vi "Autonomous Independent.vi"() -> ()   [LabVIEW 2015]
doc: "This VI is called when autonomous begins, and will automatically be terminated when autonomous ends. You can carry out timed or sensor driven robot movement independently without needing to return to the caller."
uses:
  <vilib>/Rock Robotics/WPI/Utilities/WPI_GetSetVariantRefNum.vi
  <vilib>/Rock Robotics/Network Tables/NT Read String.vi
  <vilib>/Rock Robotics/Network Tables/NT Write Numeric Array.vi
  <vilib>/Rock Robotics/Network Tables/NT Write Number.vi
  <vilib>/addons/control/pid/pid.llb/PID (DBL).vi
  Robot Global Data.vi
  <vilib>/Rock Robotics/Network Tables/NT Read Number.vi
  <vilib>/addons/control/pid/NI_PID_pid.lvlib
  navX Library v2/navX Library v2.lvlib
panel:
  in  "Roll":dbl
  in  "Angle":dbl
  in  "Distance":dbl=120.0
  in  "Task":u16(ring) items=["Forward", "Backward", "Turn", "Shoot", "Turn Angle", "Roll G", "Roll L"]
  in  "Aiming Gains":T1={"proportional gain (Kc)"=1.0, "integral time (Ti, min)"=0.01, "derivative time (Td, min)"=0.0} {"derivative time (Td, min)" format="%.3f"; "integral time (Ti, min)" format="%.3f"; "proportional gain (Kc)" format="%.3f"}
  out "Yaw":dbl(graph)
  in  "Target Angle":dbl=30.0
  out "E1 Rate":dbl
  out "E2 Rate":dbl
  out "Yaw Display":dbl
  in  "Single Turn Gains":T1={"proportional gain (Kc)"=0.12, "integral time (Ti, min)"=0.0, "derivative time (Td, min)"=0.0} {"derivative time (Td, min)" format="%.3f"; "integral time (Ti, min)" format="%.3f"; "proportional gain (Kc)" format="%.3f"}
  in  "Yaw":T1={"proportional gain (Kc)"=0.2, "integral time (Ti, min)"=0.0, "derivative time (Td, min)"=0.0} {"derivative time (Td, min)" format="%.3f"; "integral time (Ti, min)" format="%.3f"; "proportional gain (Kc)" format="%.3f"}
  out "Right Motor Speed":dbl(graph)
  out "Left Motor Speed":dbl(graph)
  out "Right Motor":dbl(graph)
  out "Left Motor":dbl(graph)
  in  "Distance":dbl=120.0
  in  "Speed Gains":T1={"proportional gain (Kc)"=0.65, "integral time (Ti, min)"=0.001, "derivative time (Td, min)"=0.001} {"derivative time (Td, min)" format="%.3f"; "integral time (Ti, min)" format="%.3f"; "proportional gain (Kc)" format="%.3f"}
  out "E2 Dist":dbl
  out "E1 Dist":dbl
  # "Be sure to right-click and choose Data Operations>>Make Current Value default if you want to save the array values with the VI"
  # "Encoder Distance Traveled"
  # "Speed we are assigning the motors and Encoder Rate"
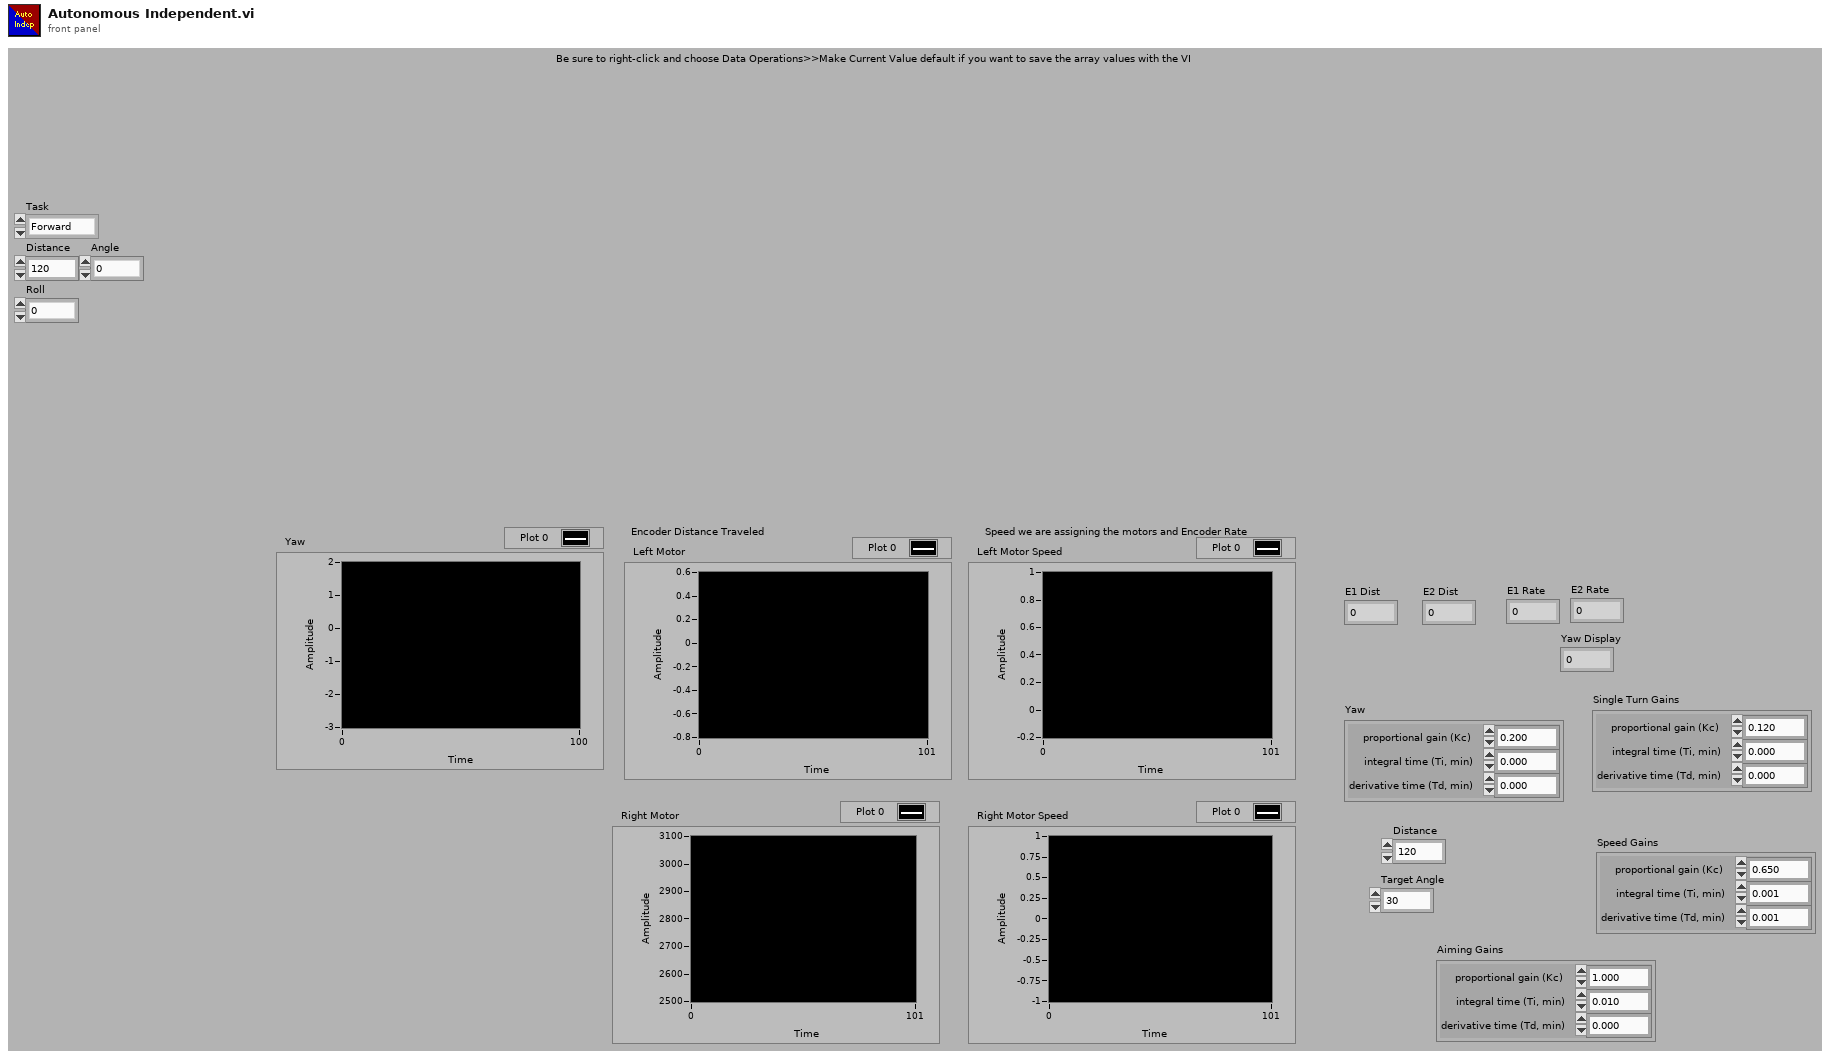
[diagram p1: front panel]
types:
  T1 = cluster{"proportional gain (Kc)":dbl, "integral time (Ti, min)":dbl, "derivative time (Td, min)":dbl}
  T2 = typedef "WPI_JoystickDevRef.ctl" = cluster{"Device":T3}
  T3 = typedef "WPI_JoystickDeviceEnum.ctl" = enum16{"USB 0", "USB 1", "USB 2", "USB 3", "USB 4", "USB 5"}
  T4 = typedef "navX Library v2.lvlib/Z900_navX_DeviceTypeDef.ctl" = cluster{"Interface":cluster{"Protocol":T5, "Update Rate (4Hz-60Hz)":u8, "navX Open TypeDef":variant}, "Notify Packet":refnum<notifier>, "Loop VI Refnum":refnum<vi>, "Ready to Close Occurrence Refnum":refnum<k4>}
  T5 = typedef "navX Library v2.lvlib/Z900_navX_ProtocolTypeDef.ctl" = enum16{"SERIAL", "I2C", "SPI"}
  T6 = typedef "WPI_EncoderDevRef.ctl" = cluster{"DevStatus":errorcluster, "EncoderIndex":T7, "CounterIndex":T8, "DistancePerCount":dbl, "Decoding Type":T9}
  T7 = typedef "FPGA_EncoderIdx.ctl" = enum8{"Enc 0", "Enc 1", "Enc 2", "Enc 3", "Enc 4", "Enc 5", "Enc 6", "Enc 7", "Invalid"}
  T8 = typedef "FPGA_CounterCtrSystemIndex.ctl" = enum8{"Ctr 0", "Ctr 1", "Ctr 2", "Ctr 3", "Ctr 4", "Ctr 5", "Ctr 6", "Ctr 7", "Invalid"}
  T9 = typedef "WPI_EncoderType.ctl" = enum16{"1x", "2x", "4x"}
  T10 = cluster{"Yaw":dbl, "Roll":dbl, "Pitch":dbl, "Heading":dbl, "Fused Heading":dbl}
  T11 = typedef "WPI_RobotDriveDevRef.ctl" = cluster{"DevStatus":errorcluster, "Motors[]":T12[], "Square Inputs":bool, "Max Output":dbl}
  T12 = typedef "WPI_MotorControlDeviceRef.ctl" = cluster{"DeviceStatus":errorcluster, "Type":T13, "PWM":cluster{"PWM Channel":T14, "DeadBand":T15}, "CAN":cluster{"Device Number":u8, "Control Mode":T16, "Semaphore":T17, "Max Vout":dbl, "TalonSRX Control Mode":T18}, "Invert":bool}
  T13 = typedef "WPI_MotorControlType.ctl" = enum16{"PWM", "CAN", "CANTalonSRX"}
  T14 = typedef "FPGA_DIOPWMChannel.ctl" = enum8{"PWM 0", "PWM 1", "PWM 2", "PWM 3", "PWM 4", "PWM 5", "PWM 6", "PWM 7", "PWM 8", "PWM 9", "PWM MXP 0", "PWM MXP 1", "PWM MXP 2", "PWM MXP 3", "PWM MXP 4", "PWM MXP 5", "PWM MXP 6", "PWM MXP 7", "PWM MXP 8", "PWM MXP 9", "Invalid"}
  T15 = typedef "WPI_PWMDeadband.ctl" = cluster{"Name":string, "maxPositivePwm":i32, "minPositivePwm":i32, "centerPwm":i32, "maxNegativePwm":i32, "minNegativePwm":i32, "angularRange":u16}
  T16 = typedef "WPI_CANJaguar_ControlMode.ctl" = enum8{"Percent VBus", "Current", "Speed", "Position", "Voltage"}
  T17 = typedef "Semaphore RefNum" = refnum<k1>
  T18 = typedef "WPI_CANTalonSRX_APIControlMode.ctl" = enum8{"Percent VBus", "Speed", "Position", "Slave", "Unchanged / Invalid", "Voltage Compensation", "Current", "Motion Profile"}
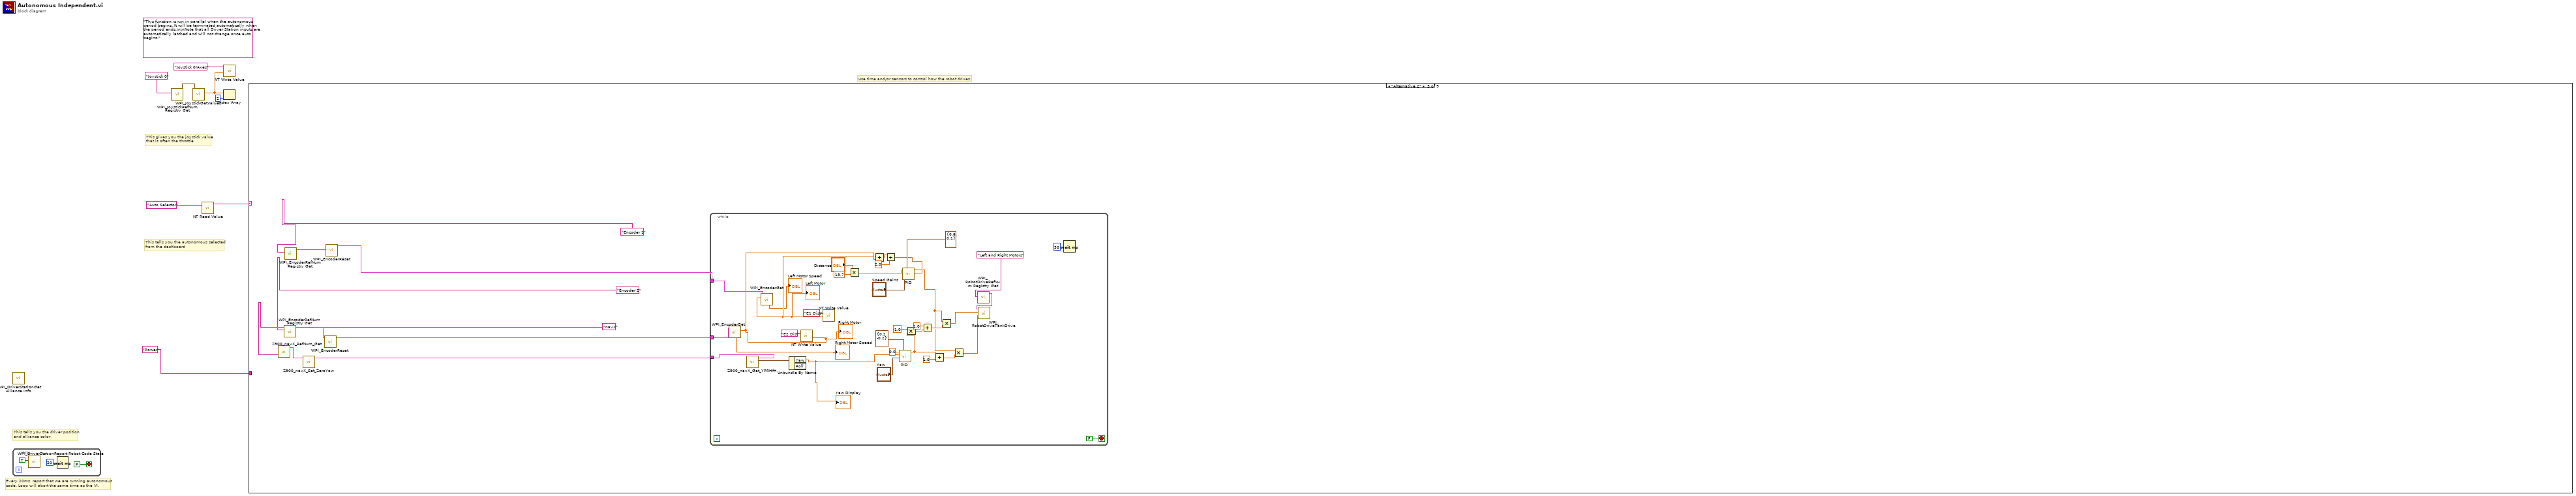
[diagram p0: block diagram]
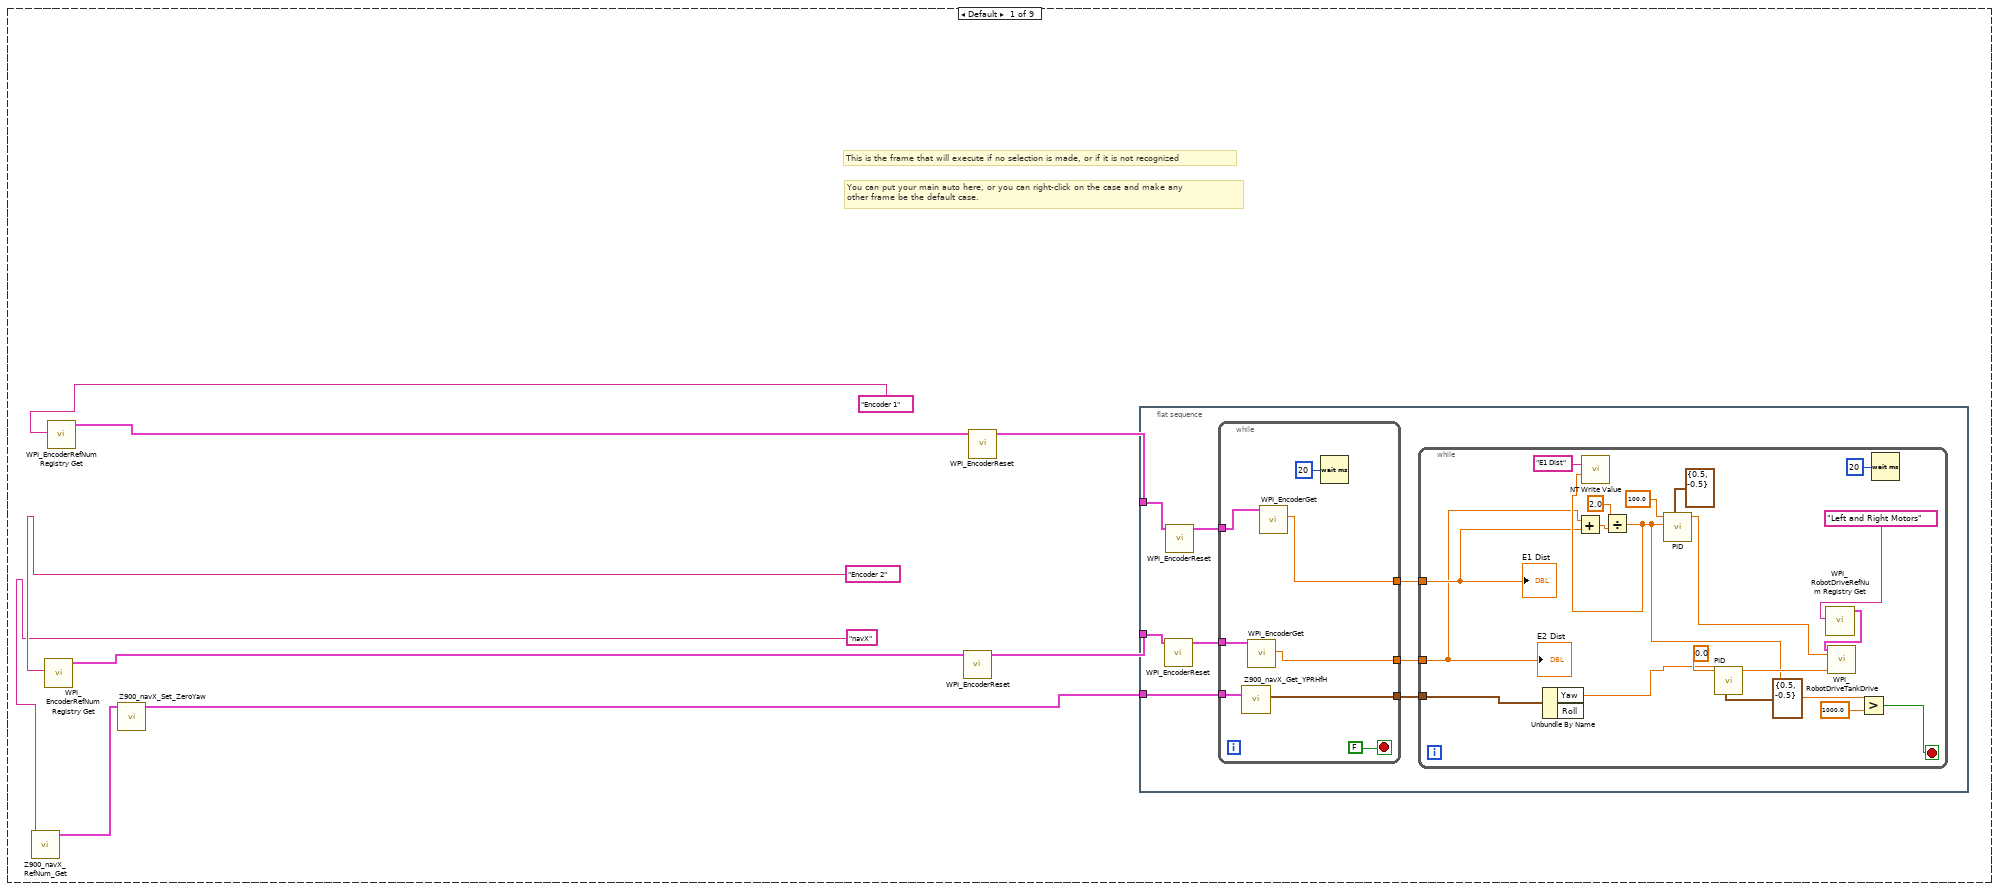
[diagram p2: hidden frame]
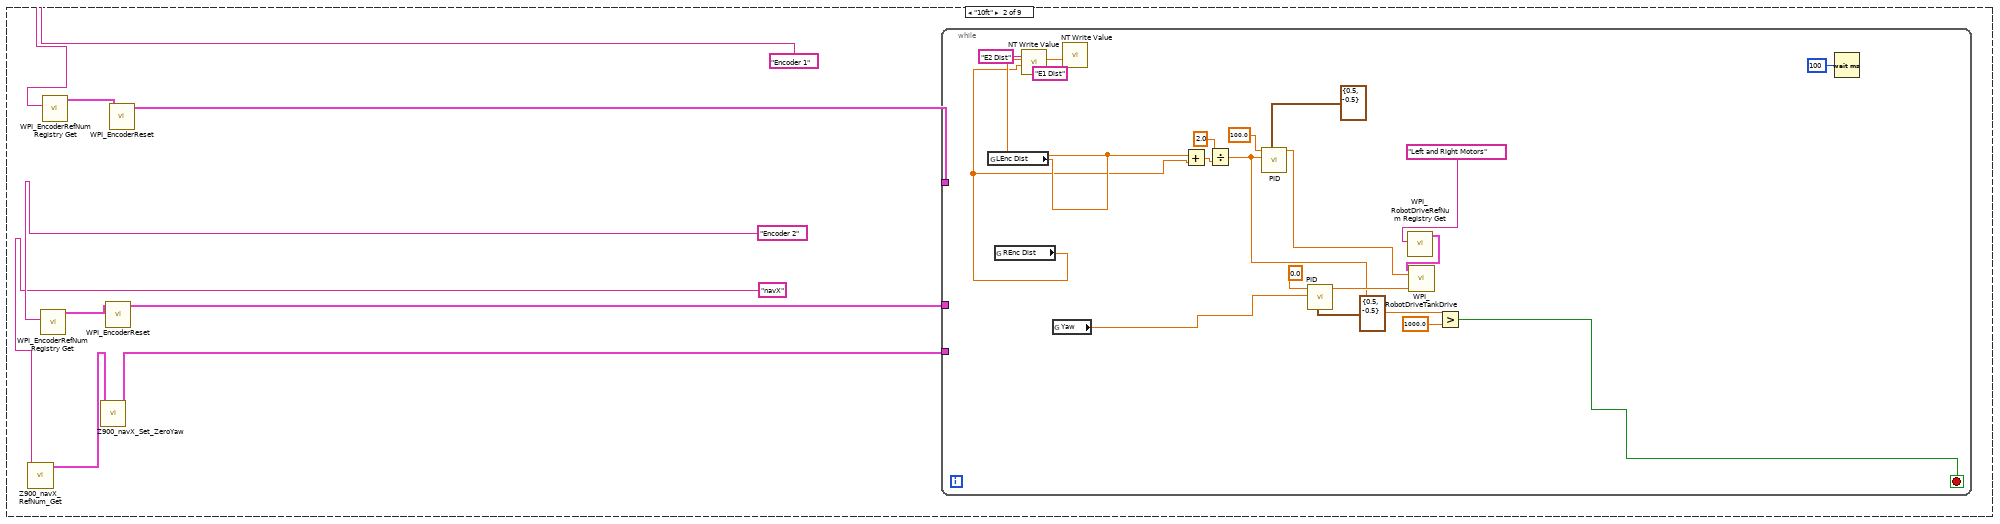
[diagram p3: hidden frame]
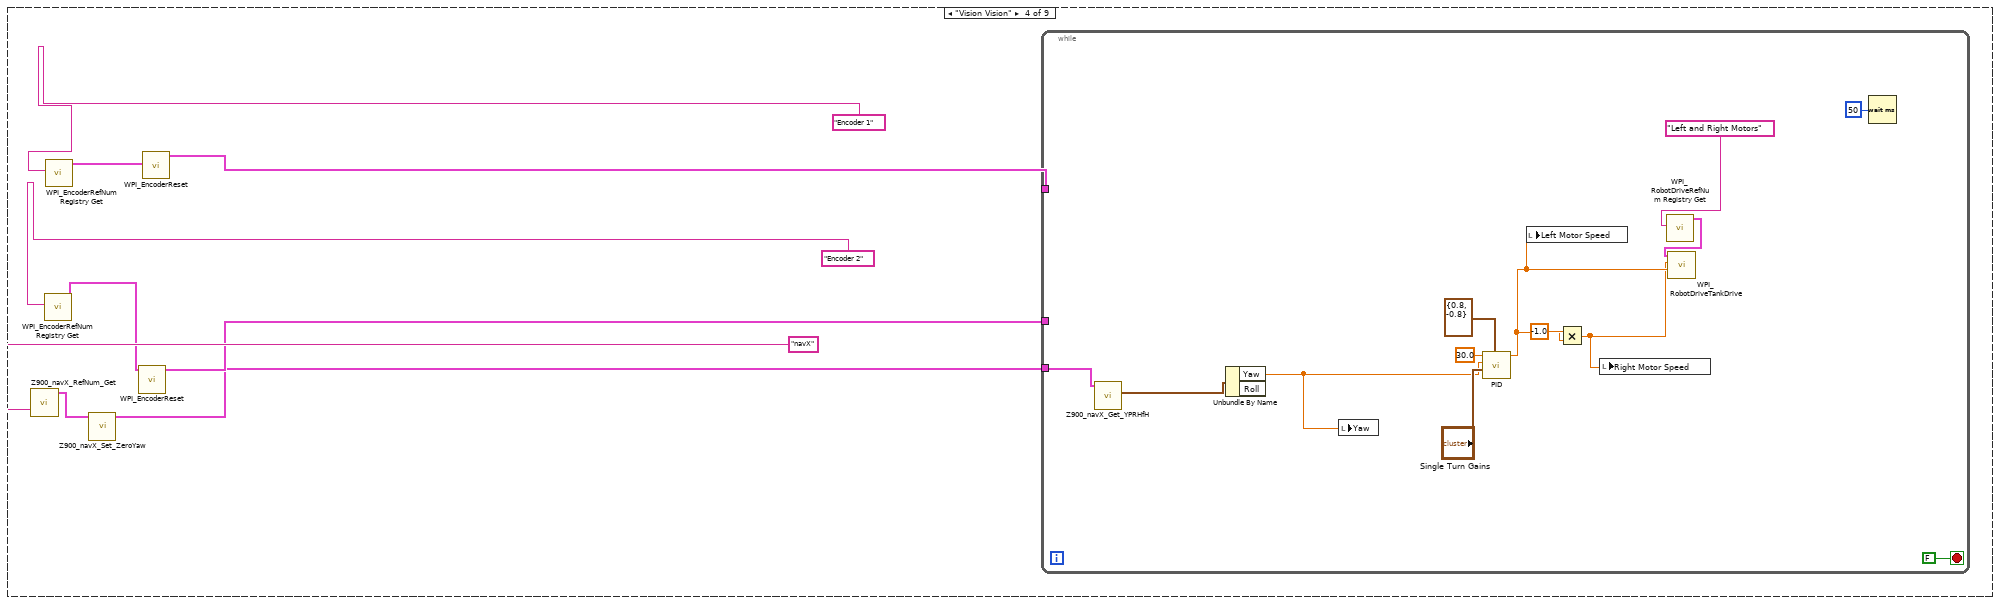
[diagram p4: hidden frame]
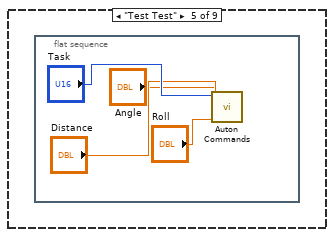
[diagram p5: hidden frame]
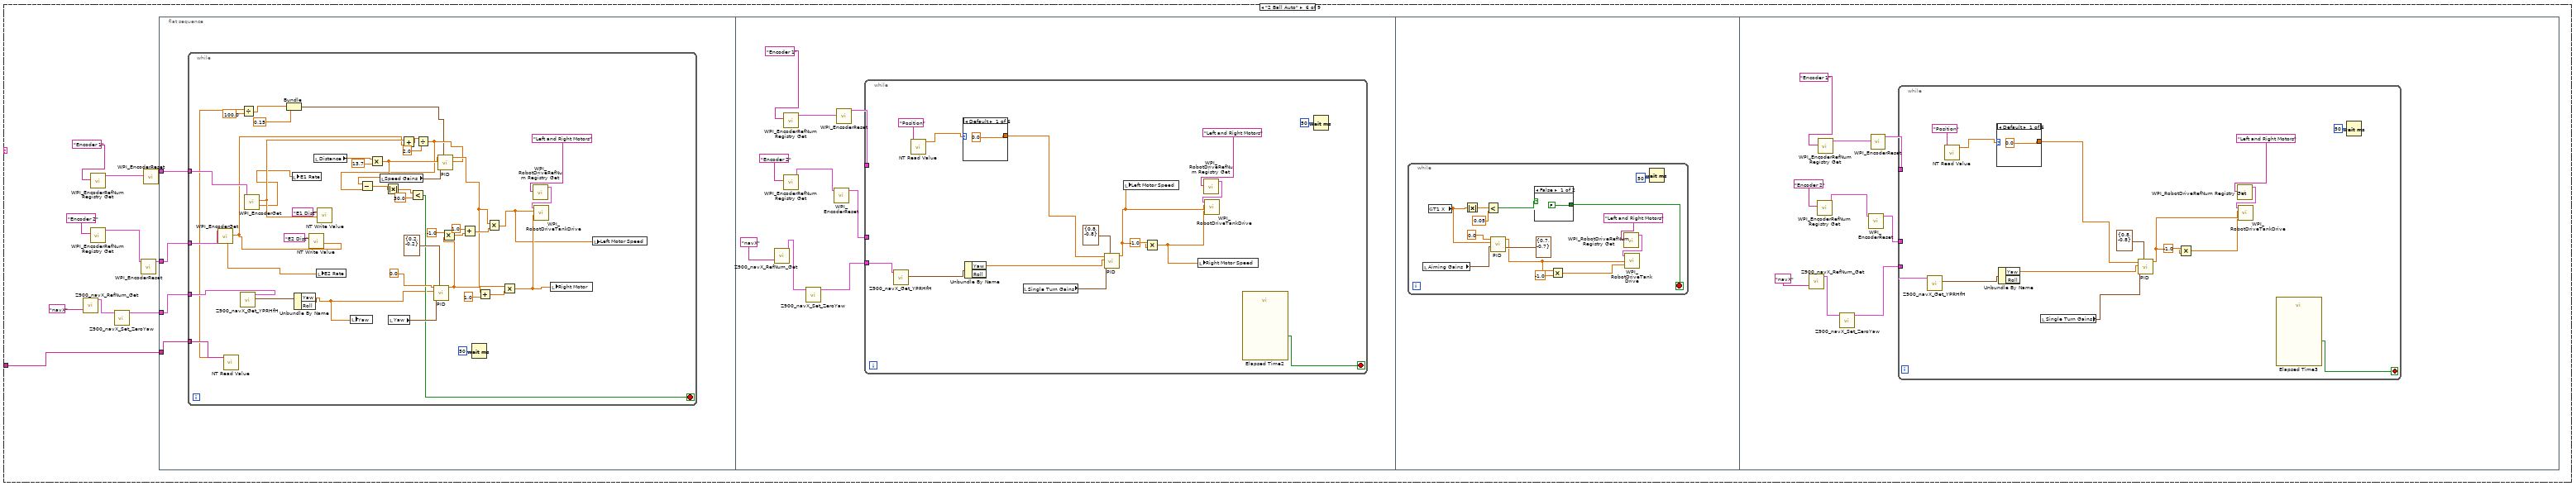
[diagram p6: hidden frame]
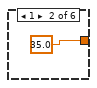
[diagram p7: hidden frame]
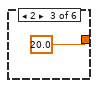
[diagram p8: hidden frame]
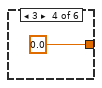
[diagram p9: hidden frame]
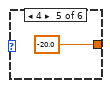
[diagram p10: hidden frame]
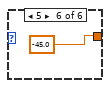
[diagram p11: hidden frame]
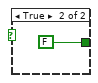
[diagram p12: hidden frame]
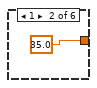
[diagram p13: hidden frame]
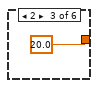
[diagram p14: hidden frame]
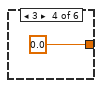
[diagram p15: hidden frame]
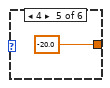
[diagram p16: hidden frame]
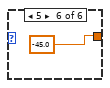
[diagram p17: hidden frame]
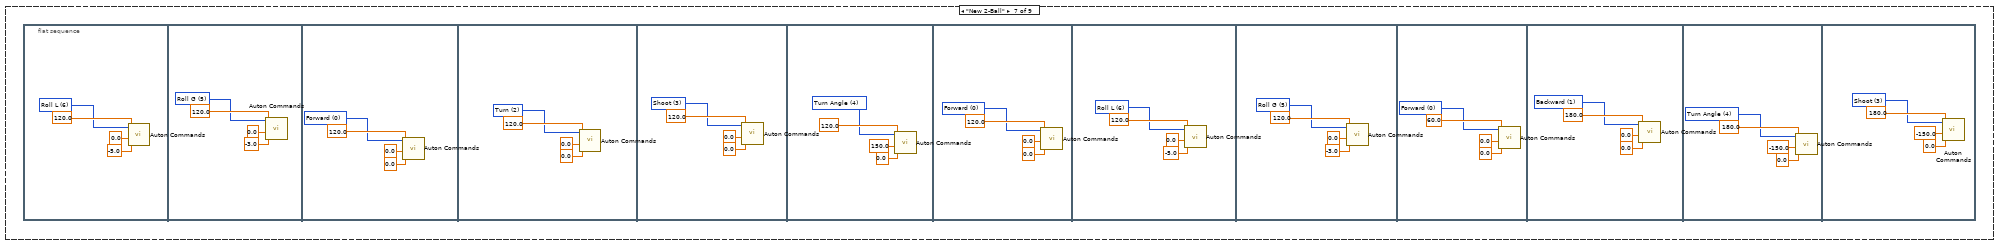
[diagram p18: hidden frame]
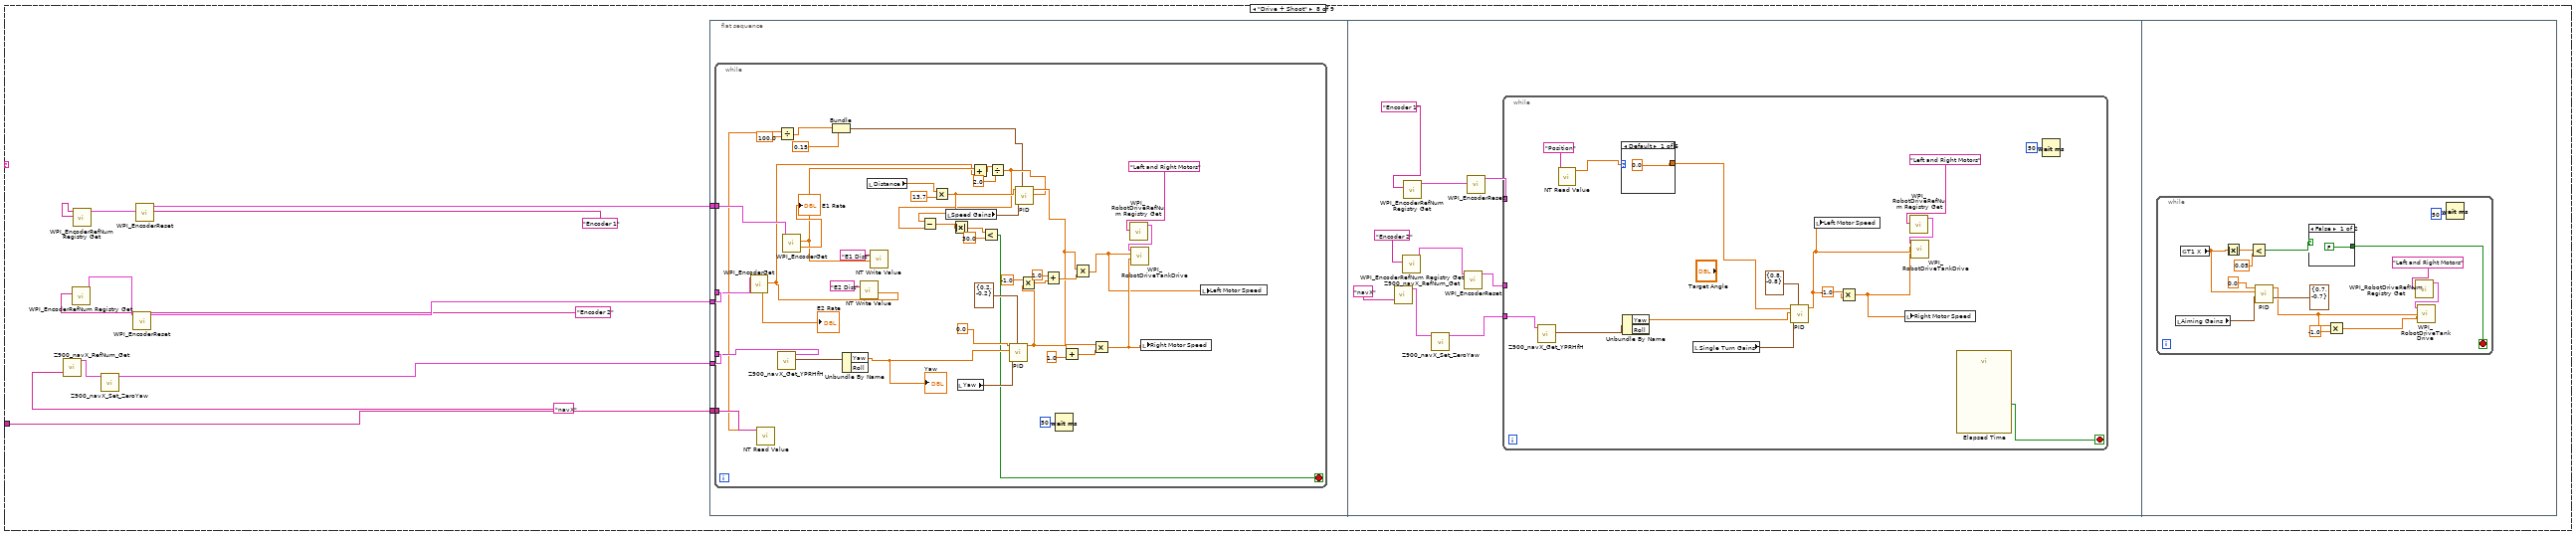
[diagram p19: hidden frame]
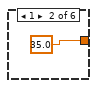
[diagram p20: hidden frame]
diagram:
  (unwired) "This function is run in parallel when the autonomous period begins. It will be terminated automatically when the period ends.\n\nNote that all Driver Station inputs are automatically latched and will not change once auto begins."
  # "This tells you the autonomous selected\nfrom the dashboard"
  # "Every 20ms, report that we are running autonomous\ncode. Loop will abort the same time as the VI."
  # "This gives you the joystick value\nthat is often the throttle"
  # "Use time and/or sensors to control how the robot drives."
  # "This tells you the driver position\nand alliance color"
  n1 = while {
    stop <- FALSE stop-if-true
    n2 = call <vilib>:"WPI_DriverStationReport Robot Code State.vi"("Autonomous"=TRUE) -> ()  [unwired: 10 in, 1 out]
    n3 = Wait (ms)(milliseconds to wait=u32 20) -> ()  [unwired: 1 out]
  }
  n4 = call <vilib>:"WPI_DriverStationGet Alliance Info.vi"() -> ()  [unwired: 12 out]
  n5 = call <vilib>:"WPI_JoystickRefNum Registry Get.vi"("refnum name"="Joystick 0") -> ("JoystickDevRef"=w7:T2)  [unwired: 1 in, 9 out]
  n6 = call <vilib>:"WPI_JoystickGetValues.vi"("JoystickDevRef"=w7) -> ("Axes"=w3:dbl[])  [unwired: 6 in, 4 out]
  n7 = call-poly <vilib>:"NT Read Value.vi"("Name"="Auto Selector") -> ("String"=w4:string)  [unwired: 9 in, 1 out]
  n8 = call-poly <vilib>:"NT Write Value.vi"("Numeric Array"=w3, "Name"="Joystick 0/Axes") -> ()  [unwired: 9 in, 1 out]
  n9 = Index Array(array=w3, index=2) -> ()  [unwired: 1 out]
  n10 = case shown="\"Alternative 2\"" w4 {
    tunnel: "Power" ("Name") -> [_ _ _ _ _ w155 _ w341 _]
    frame Default {
      # "You can put your main auto here, or you can right-click on the case and make any\nother frame be the default case."
      # "This is the frame that will execute if no selection is made, or if it is not recognized"
      n11 = call "Z900_navX_RefNum_Get.vi"("refnum name"="navX") -> ("navX Device"=w14:T4)  [unwired: 9 in, 1 out]
      n12 = call <vilib>:"WPI_EncoderRefNum Registry Get.vi"("refnum name"="Encoder 2") -> ("EncoderDevRef"=w16:T6)  [unwired: 9 in, 1 out]
      n13 = call <vilib>:"WPI_EncoderRefNum Registry Get.vi"("refnum name"="Encoder 1") -> ("EncoderDevRef"=w18:T6)  [unwired: 9 in, 1 out]
      n14 = call "Z900_navX_Set_ZeroYaw.vi"("navX Device"=w14) -> ("navX Device"=w13:T4)  [unwired: 9 in, 1 out]
      n15 = call <vilib>:"WPI_EncoderReset.vi"("EncoderDevRef"=w16) -> ("EncoderDevRef"=w15:T6)  [unwired: 9 in, 1 out]
      n16 = call <vilib>:"WPI_EncoderReset.vi"("EncoderDevRef"=w18) -> ("EncoderDevRef"=w17:T6)  [unwired: 9 in, 1 out]
      n17 = flat-sequence {
        tunnel: w17 -> [w28]
        tunnel: w15 -> [w27]
        tunnel: w13 -> [w26]
        frame #0 {
          n18 = call <vilib>:"WPI_EncoderReset.vi"("EncoderDevRef"=w27) -> ("EncoderDevRef"=w25:T6)  [unwired: 9 in, 1 out]
          n19 = call <vilib>:"WPI_EncoderReset.vi"("EncoderDevRef"=w28) -> ("EncoderDevRef"=w24:T6)  [unwired: 9 in, 1 out]
          n20 = while {
            tunnel: w26 -> [w33]
            tunnel: w25 -> [w34]
            tunnel: w24 -> [w35]
            tunnel: [w32] -> w23
            tunnel: [w31] -> w22
            tunnel: [w30] -> w21
            stop <- FALSE stop-if-true
            n21 = call "Z900_navX_Get_YPRHfH.vi"("navX Device"=w33) -> ("YRPHfH"=w32:T10)  [unwired: 7 in, 3 out]
            n22 = call <vilib>:"WPI_EncoderGet.vi"("EncoderDevRef"=w34) -> ("Distance"=w31:dbl)  [unwired: 5 in, 5 out]
            n23 = call <vilib>:"WPI_EncoderGet.vi"("EncoderDevRef"=w35) -> ("Distance"=w30:dbl)  [unwired: 5 in, 5 out]
            n24 = Wait (ms)(milliseconds to wait=u32 20) -> ()  [unwired: 1 out]
          }
          n25 = while {
            tunnel: w23 -> [w40]
            tunnel: w22 -> [w38]
            tunnel: w21 -> [w39]
            stop <- w44 stop-if-true
            n26 = Unbundle By Name(w40) -> ("Yaw"=w41:dbl)  [unwired: 1 out]
            n27 = Add(x=w38, y=w39) -> (x+y=w55:dbl)
            n28 = Divide(x=2.0, y=w55) -> (x/y=w43:dbl)
            n29 = call-poly <vilib>:"NT Write Value.vi"("Numeric"=w43, "Name"="E1 Dist") -> ()  [unwired: 9 in, 1 out]
            n30 = call-poly <vilib>:"PID.vi"("output range"=cluster{"output high":dbl, "output low":dbl} {"output high"=0.5, "output low"=-0.5}, "process variable"=w43, "setpoint"=100.0) -> ("output"=w48:dbl)  [unwired: 7 in, 1 out]
            n31 = call-poly <vilib>:"PID.vi"("output range"=cluster{"output high":dbl, "output low":dbl} {"output high"=0.5, "output low"=-0.5}, "process variable"=w41, "setpoint"=0.0) -> ("output"=w47:dbl)  [unwired: 7 in, 1 out]
            n32 = call <vilib>:"WPI_RobotDriveRefNum Registry Get.vi"("refnum name"="Left and Right Motors") -> ("RobotDriveDevRef"=w50:T11)  [unwired: 9 in, 1 out]
            n33 = call <vilib>:"WPI_RobotDriveTankDrive.vi"("Right axis value"=w47, "Left axis value"=w48, "RobotDriveDevRef"=w50) -> ()  [unwired: 6 in, 3 out]
            n34 = Greater?(x=w43, y=1000.0) -> (0:w44:bool)
            n35 = Wait (ms)(milliseconds to wait=u32 20) -> ()  [unwired: 1 out]
            "E2 Dist" <- w38
            "E1 Dist" <- w39
          }
        }
      }
    }
    frame "10ft" {
      n36 = call "Z900_navX_RefNum_Get.vi"("refnum name"="navX") -> ("navX Device"=w58:T4)  [unwired: 9 in, 1 out]
      n37 = call <vilib>:"WPI_EncoderRefNum Registry Get.vi"("refnum name"="Encoder 2") -> ("EncoderDevRef"=w60:T6)  [unwired: 9 in, 1 out]
      n38 = call <vilib>:"WPI_EncoderRefNum Registry Get.vi"("refnum name"="Encoder 1") -> ("EncoderDevRef"=w62:T6)  [unwired: 9 in, 1 out]
      n39 = call "Z900_navX_Set_ZeroYaw.vi"("navX Device"=w58) -> ("navX Device"=w57:T4)  [unwired: 9 in, 1 out]
      n40 = call <vilib>:"WPI_EncoderReset.vi"("EncoderDevRef"=w60) -> ("EncoderDevRef"=w59:T6)  [unwired: 9 in, 1 out]
      n41 = call <vilib>:"WPI_EncoderReset.vi"("EncoderDevRef"=w62) -> ("EncoderDevRef"=w61:T6)  [unwired: 9 in, 1 out]
      n42 = while {
        tunnel: w61 -> [_]
        tunnel: w59 -> [_]
        tunnel: w57 -> [_]
        stop <- w65 stop-if-true
        n43 = global read "Robot Global Data.vi" "LEnc Dist"() -> (w68:dbl)
        n44 = global read "Robot Global Data.vi" "REnc Dist"() -> (w67:dbl)
        n45 = call-poly <vilib>:"NT Write Value.vi"("Numeric"=w67, "Name"="E2 Dist") -> ()  [unwired: 9 in, 1 out]
        n46 = global read "Robot Global Data.vi" "Yaw"() -> (w66:dbl)
        n47 = call-poly <vilib>:"NT Write Value.vi"("Numeric"=w68, "Name"="E1 Dist") -> ()  [unwired: 9 in, 1 out]
        n48 = Add(x=w68, y=w67) -> (x+y=w82:dbl)
        n49 = Divide(x=2.0, y=w82) -> (x/y=w72:dbl)
        n50 = call-poly <vilib>:"PID.vi"("output range"=cluster{"output high":dbl, "output low":dbl} {"output high"=0.5, "output low"=-0.5}, "process variable"=w72, "setpoint"=100.0) -> ("output"=w76:dbl)  [unwired: 7 in, 1 out]
        n51 = call-poly <vilib>:"PID.vi"("output range"=cluster{"output high":dbl, "output low":dbl} {"output high"=0.5, "output low"=-0.5}, "process variable"=w66, "setpoint"=0.0) -> ("output"=w75:dbl)  [unwired: 7 in, 1 out]
        n52 = call <vilib>:"WPI_RobotDriveRefNum Registry Get.vi"("refnum name"="Left and Right Motors") -> ("RobotDriveDevRef"=w78:T11)  [unwired: 9 in, 1 out]
        n53 = call <vilib>:"WPI_RobotDriveTankDrive.vi"("Right axis value"=w75, "Left axis value"=w76, "RobotDriveDevRef"=w78) -> ()  [unwired: 6 in, 3 out]
        n54 = Greater?(x=w72, y=1000.0) -> (0:w65:bool)
        n55 = Wait (ms)(milliseconds to wait=u32 100) -> ()  [unwired: 1 out]
      }
    }
    frame "Alternative 2" {
      n56 = call "Z900_navX_RefNum_Get.vi"("refnum name"="navX") -> ("navX Device"=w85:T4)  [unwired: 9 in, 1 out]
      n57 = call <vilib>:"WPI_EncoderRefNum Registry Get.vi"("refnum name"="Encoder 2") -> ("EncoderDevRef"=w87:T6)  [unwired: 9 in, 1 out]
      n58 = call <vilib>:"WPI_EncoderRefNum Registry Get.vi"("refnum name"="Encoder 1") -> ("EncoderDevRef"=w89:T6)  [unwired: 9 in, 1 out]
      n59 = call "Z900_navX_Set_ZeroYaw.vi"("navX Device"=w85) -> ("navX Device"=w84:T4)  [unwired: 9 in, 1 out]
      n60 = call <vilib>:"WPI_EncoderReset.vi"("EncoderDevRef"=w87) -> ("EncoderDevRef"=w86:T6)  [unwired: 9 in, 1 out]
      n61 = call <vilib>:"WPI_EncoderReset.vi"("EncoderDevRef"=w89) -> ("EncoderDevRef"=w88:T6)  [unwired: 9 in, 1 out]
      n62 = while {
        tunnel: w88 -> [w121]
        tunnel: w86 -> [w120]
        tunnel: w84 -> [w119]
        stop <- FALSE stop-if-true
        n63 = call <vilib>:"WPI_EncoderGet.vi"("EncoderDevRef"=w120) -> ("Distance"=w110:dbl, "Rate"=→"Right Motor Speed":dbl)  [unwired: 5 in, 4 out]
        "Right Motor" <- w110
        n64 = call "Z900_navX_Get_YPRHfH.vi"("navX Device"=w119) -> ("YRPHfH"=w122:T10)  [unwired: 7 in, 3 out]
        n65 = call <vilib>:"WPI_EncoderGet.vi"("EncoderDevRef"=w121) -> ("Distance"=w109:dbl, "Rate"=→"Left Motor Speed":dbl)  [unwired: 5 in, 4 out]
        "Left Motor" <- w109
        n66 = Unbundle By Name(w122) -> ("Yaw"=w95:dbl)  [unwired: 1 out]
        "Yaw Display" <- w95
        n67 = call-poly <vilib>:"NT Write Value.vi"("Numeric"=w110, "Name"="E2 Dist") -> ()  [unwired: 9 in, 1 out]
        n68 = call-poly <vilib>:"NT Write Value.vi"("Numeric"=w109, "Name"="E1 Dist") -> ()  [unwired: 9 in, 1 out]
        n69 = Multiply(x="Distance", y=13.7) -> (x*y=w111:dbl)
        n70 = Add(x=w109, y=w110) -> (x+y=w116:dbl)
        n71 = Divide(x=w116, y=2.0) -> (x/y=w114:dbl)
        n72 = call-poly <vilib>:"PID.vi"("output range"=cluster{"output high":dbl, "output low":dbl} {"output high"=0.2, "output low"=-0.2}, "PID gains"="Yaw", "process variable"=w95, "setpoint"=0.0) -> ("output"=w99:dbl)  [unwired: 6 in, 1 out]
        n73 = call-poly <vilib>:"PID.vi"("output range"=cluster{"output high":dbl, "output low":dbl} {"output high"=0.6, "output low"=0.1}, "PID gains"="Speed Gains", "process variable"=w114, "setpoint"=w111) -> ("output"=w96:dbl)  [unwired: 6 in, 1 out]
        n74 = Multiply(x=-1.0, y=w99) -> (x*y=w100:dbl)
        n75 = Add(x=1.0, y=w100) -> (x+y=w101:dbl)
        n76 = Add(x=w99, y=1.0) -> (x+y=w102:dbl)
        n77 = Multiply(x=w96, y=w101) -> (x*y=w93:dbl)
        n78 = Multiply(x=w96, y=w102) -> (x*y=w94:dbl)
        n79 = call <vilib>:"WPI_RobotDriveRefNum Registry Get.vi"("refnum name"="Left and Right Motors") -> ("RobotDriveDevRef"=w124:T11)  [unwired: 9 in, 1 out]
        n80 = call <vilib>:"WPI_RobotDriveTankDrive.vi"("Right axis value"=w94, "Left axis value"=w93, "RobotDriveDevRef"=w124) -> ()  [unwired: 6 in, 3 out]
        n81 = Wait (ms)(milliseconds to wait=u32 50) -> ()  [unwired: 1 out]
      }
    }
    frame "Vision Vision" {
      n82 = call "Z900_navX_RefNum_Get.vi"("refnum name"="navX") -> ("navX Device"=w130:T4)  [unwired: 9 in, 1 out]
      n83 = call <vilib>:"WPI_EncoderRefNum Registry Get.vi"("refnum name"="Encoder 2") -> ("EncoderDevRef"=w132:T6)  [unwired: 9 in, 1 out]
      n84 = call <vilib>:"WPI_EncoderRefNum Registry Get.vi"("refnum name"="Encoder 1") -> ("EncoderDevRef"=w134:T6)  [unwired: 9 in, 1 out]
      n85 = call "Z900_navX_Set_ZeroYaw.vi"("navX Device"=w130) -> ("navX Device"=w129:T4)  [unwired: 9 in, 1 out]
      n86 = call <vilib>:"WPI_EncoderReset.vi"("EncoderDevRef"=w132) -> ("EncoderDevRef"=w131:T6)  [unwired: 9 in, 1 out]
      n87 = call <vilib>:"WPI_EncoderReset.vi"("EncoderDevRef"=w134) -> ("EncoderDevRef"=w133:T6)  [unwired: 9 in, 1 out]
      n88 = while {
        tunnel: w133 -> [_]
        tunnel: w131 -> [_]
        tunnel: w129 -> [w144]
        stop <- FALSE stop-if-true
        n89 = call "Z900_navX_Get_YPRHfH.vi"("navX Device"=w144) -> ("YRPHfH"=w143:T10)  [unwired: 7 in, 3 out]
        n90 = Unbundle By Name(w143) -> ("Yaw"=w138:dbl)  [unwired: 1 out]
        n91 = local write "Yaw"(w138) -> ()
        n92 = call-poly <vilib>:"PID.vi"("output range"=cluster{"output high":dbl, "output low":dbl} {"output high"=0.8, "output low"=-0.8}, "PID gains"="Single Turn Gains", "process variable"=w138, "setpoint"=30.0) -> ("output"=w140:dbl)  [unwired: 6 in, 1 out]
        n93 = local write "Left Motor Speed"(w140) -> ()
        n94 = Multiply(x=-1.0, y=w140) -> (x*y=w139:dbl)
        n95 = local write "Right Motor Speed"(w139) -> ()
        n96 = call <vilib>:"WPI_RobotDriveRefNum Registry Get.vi"("refnum name"="Left and Right Motors") -> ("RobotDriveDevRef"=w149:T11)  [unwired: 9 in, 1 out]
        n97 = call <vilib>:"WPI_RobotDriveTankDrive.vi"("Right axis value"=w140, "Left axis value"=w139, "RobotDriveDevRef"=w149) -> ()  [unwired: 6 in, 3 out]
        n98 = Wait (ms)(milliseconds to wait=u32 50) -> ()  [unwired: 1 out]
      }
    }
    frame "Test Test" {
      n99 = flat-sequence {
        frame #0 {
          n100 = call "Auton Commands.vi"("Roll"="Roll", "Turn Angle"="Angle", "Distance"="Distance", "Task"="Task") -> ()  [unwired: 7 in]
        }
      }
    }
    frame "2 Ball Auto" {
      n101 = call "Z900_navX_RefNum_Get.vi"("refnum name"="navX") -> ("navX Device"=w163:T4)  [unwired: 9 in, 1 out]
      n102 = call <vilib>:"WPI_EncoderRefNum Registry Get.vi"("refnum name"="Encoder 2") -> ("EncoderDevRef"=w161:T6)  [unwired: 9 in, 1 out]
      n103 = call <vilib>:"WPI_EncoderRefNum Registry Get.vi"("refnum name"="Encoder 1") -> ("EncoderDevRef"=w159:T6)  [unwired: 9 in, 1 out]
      n104 = call "Z900_navX_Set_ZeroYaw.vi"("navX Device"=w163) -> ("navX Device"=w164:T4)  [unwired: 9 in, 1 out]
      n105 = call <vilib>:"WPI_EncoderReset.vi"("EncoderDevRef"=w161) -> ("EncoderDevRef"=w162:T6)  [unwired: 9 in, 1 out]
      n106 = call <vilib>:"WPI_EncoderReset.vi"("EncoderDevRef"=w159) -> ("EncoderDevRef"=w160:T6)  [unwired: 9 in, 1 out]
      n107 = flat-sequence {
        tunnel: w164 -> [w168]
        tunnel: w162 -> [w167]
        tunnel: w160 -> [w166]
        tunnel: w155 -> [w165]
        frame #0 {
          n108 = while {
            tunnel: w166 -> [w206]
            tunnel: w167 -> [w205]
            tunnel: w168 -> [w204]
            tunnel: w165 -> [w178]
            stop <- w179 stop-if-true
            n109 = call <vilib>:"WPI_EncoderGet.vi"("EncoderDevRef"=w205) -> ("Distance"=w185:dbl, "Rate"=w170:dbl)  [unwired: 5 in, 4 out]
            n110 = call-poly <vilib>:"NT Read Value.vi"("Name"=w178) -> ("Numeric"=w177:dbl)  [unwired: 9 in, 1 out]
            n111 = call "Z900_navX_Get_YPRHfH.vi"("navX Device"=w204) -> ("YRPHfH"=w207:T10)  [unwired: 7 in, 3 out]
            n112 = Divide(x=w177, y=100.0) -> (x/y=w175:dbl)
            n113 = call <vilib>:"WPI_EncoderGet.vi"("EncoderDevRef"=w206) -> ("Distance"=w186:dbl, "Rate"=w169:dbl)  [unwired: 5 in, 4 out]
            n114 = Bundle(w175, "output low"=0.15) -> (w173:cluster{dbl, "output low":dbl})  [unwired: 1 in]
            n115 = local write "E1 Rate"(w169) -> ()
            n116 = Unbundle By Name(w207) -> ("Yaw"=w171:dbl)  [unwired: 1 out]
            n117 = call-poly <vilib>:"NT Write Value.vi"("Numeric"=w185, "Name"="E2 Dist") -> ()  [unwired: 9 in, 1 out]
            n118 = local read "Distance"() -> (w172:dbl)
            n119 = local write "E2 Rate"(w170) -> ()
            n120 = call-poly <vilib>:"NT Write Value.vi"("Numeric"=w186, "Name"="E1 Dist") -> ()  [unwired: 9 in, 1 out]
            n121 = local write "Yaw"(w171) -> ()
            n122 = Multiply(x=w172, y=13.7) -> (x*y=w184:dbl)
            n123 = local read "Speed Gains"() -> (w188:T1)
            n124 = local read "Yaw"() -> (w191:T1)
            n125 = Add(x=w186, y=w185) -> (x+y=w203:dbl)
            n126 = Divide(x=w203, y=2.0) -> (x/y=w183:dbl)
            n127 = Subtract(x=w184, y=w183) -> (x-y=w182:dbl)
            n128 = Absolute Value(x=w182) -> (abs(x)=w181:dbl)
            n129 = Less?(x=w181, y=30.0) -> (x < y?=w179:bool)
            n130 = call-poly <vilib>:"PID.vi"("output range"=cluster{"output high":dbl, "output low":dbl} {"output high"=0.2, "output low"=-0.2}, "PID gains"=w191, "process variable"=w171, "setpoint"=0.0) -> ("output"=w196:dbl)  [unwired: 6 in, 1 out]
            n131 = call-poly <vilib>:"PID.vi"("output range"=w173, "PID gains"=w188, "process variable"=w183, "setpoint"=w184) -> ("output"=w193:dbl)  [unwired: 6 in, 1 out]
            n132 = Multiply(x=-1.0, y=w196) -> (x*y=w197:dbl)
            n133 = Add(x=1.0, y=w197) -> (x+y=w198:dbl)
            n134 = Wait (ms)(milliseconds to wait=u32 50) -> ()  [unwired: 1 out]
            n135 = Add(x=w196, y=1.0) -> (x+y=w199:dbl)
            n136 = Multiply(x=w193, y=w198) -> (x*y=w189:dbl)
            n137 = Multiply(x=w193, y=w199) -> (x*y=w190:dbl)
            n138 = call <vilib>:"WPI_RobotDriveRefNum Registry Get.vi"("refnum name"="Left and Right Motors") -> ("RobotDriveDevRef"=w209:T11)  [unwired: 9 in, 1 out]
            n139 = call <vilib>:"WPI_RobotDriveTankDrive.vi"("Right axis value"=w190, "Left axis value"=w189, "RobotDriveDevRef"=w209) -> ()  [unwired: 6 in, 3 out]
            n140 = local write "Right Motor"(w190) -> ()
            n141 = local write "Left Motor Speed"(w189) -> ()
          }
        }
        frame #1 {
          n142 = call "Z900_navX_RefNum_Get.vi"("refnum name"="navX") -> ("navX Device"=w214:T4)  [unwired: 9 in, 1 out]
          n143 = call <vilib>:"WPI_EncoderRefNum Registry Get.vi"("refnum name"="Encoder 2") -> ("EncoderDevRef"=w216:T6)  [unwired: 9 in, 1 out]
          n144 = call <vilib>:"WPI_EncoderRefNum Registry Get.vi"("refnum name"="Encoder 1") -> ("EncoderDevRef"=w218:T6)  [unwired: 9 in, 1 out]
          n145 = call "Z900_navX_Set_ZeroYaw.vi"("navX Device"=w214) -> ("navX Device"=w213:T4)  [unwired: 9 in, 1 out]
          n146 = call <vilib>:"WPI_EncoderReset.vi"("EncoderDevRef"=w216) -> ("EncoderDevRef"=w215:T6)  [unwired: 9 in, 1 out]
          n147 = call <vilib>:"WPI_EncoderReset.vi"("EncoderDevRef"=w218) -> ("EncoderDevRef"=w217:T6)  [unwired: 9 in, 1 out]
          n148 = while {
            tunnel: w217 -> [_]
            tunnel: w215 -> [_]
            tunnel: w213 -> [w232]
            stop <- w225 stop-if-true
            n149 = call "Z900_navX_Get_YPRHfH.vi"("navX Device"=w232) -> ("YRPHfH"=w231:T10)  [unwired: 7 in, 3 out]
            n150 = call-poly <vilib>:"NT Read Value.vi"("Name"="Position") -> ("Numeric"=w222:dbl)  [unwired: 9 in, 1 out]
            n151 = case shown="Default" w222 {
              tunnel: [0.0 35.0 20.0 0.0 -20.0 -45.0] -> w223
              frame Default {
              }
              frame 1 {
              }
              frame 2 {
              }
              frame 3 {
              }
              frame 4 {
              }
              frame 5 {
              }
            }
            n152 = Unbundle By Name(w231) -> ("Yaw"=w229:dbl)  [unwired: 1 out]
            n153 = local read "Single Turn Gains"() -> (w228:T1)
            n154 = call-poly <vilib>:"PID.vi"("output range"=cluster{"output high":dbl, "output low":dbl} {"output high"=0.8, "output low"=-0.8}, "PID gains"=w228, "process variable"=w229, "setpoint"=w223) -> ("output"=w227:dbl)  [unwired: 6 in, 1 out]
            n155 = local write "Left Motor Speed"(w227) -> ()
            n156 = Multiply(x=-1.0, y=w227) -> (x*y=w226:dbl)
            n157 = local write "Right Motor Speed"(w226) -> ()
            n158 = call <vilib>:"WPI_RobotDriveRefNum Registry Get.vi"("refnum name"="Left and Right Motors") -> ("RobotDriveDevRef"=w235:T11)  [unwired: 9 in, 1 out]
            n159 = call <vilib>:"WPI_RobotDriveTankDrive.vi"("Right axis value"=w227, "Left axis value"=w226, "RobotDriveDevRef"=w235) -> ()  [unwired: 6 in, 3 out]
            n160 = call "Elapsed Time2"() -> ("Time has Elapsed"=w225:bool)  [unwired: 12 in, 7 out]
            n161 = Wait (ms)(milliseconds to wait=u32 50) -> ()  [unwired: 1 out]
          }
        }
        frame #2 {
          n162 = while {
            stop <- w253 stop-if-true
            n163 = local read "Aiming Gains"() -> (w243:T1)
            n164 = global read "Robot Global Data.vi" "T1 X"() -> (w251:dbl)
            n165 = Absolute Value(x=w251) -> (abs(x)=w256:dbl)
            n166 = Less?(x=w256, y=0.05) -> (x < y?=w254:bool)
            n167 = call-poly <vilib>:"PID.vi"("output range"=cluster{"output high":dbl, "output low":dbl} {"output high"=0.7, "output low"=-0.7}, "PID gains"=w243, "process variable"=w251, "setpoint"=0.0) -> ("output"=w245:dbl)  [unwired: 6 in, 1 out]
            n168 = case shown="False" w254 {
              tunnel: [FALSE FALSE] -> w253
              frame False {
              }
              frame True {
              }
            }
            n169 = Multiply(x=w245, y=-1.0) -> (x*y=w244:dbl)
            n170 = call <vilib>:"WPI_RobotDriveRefNum Registry Get.vi"("refnum name"="Left and Right Motors") -> ("RobotDriveDevRef"=w247:T11)  [unwired: 9 in, 1 out]
            n171 = call <vilib>:"WPI_RobotDriveTankDrive.vi"("Right axis value"=w244, "Left axis value"=w245, "RobotDriveDevRef"=w247) -> ()  [unwired: 6 in, 3 out]
            n172 = Wait (ms)(milliseconds to wait=u32 50) -> ()  [unwired: 1 out]
          }
        }
        frame #3 {
          n173 = call "Z900_navX_RefNum_Get.vi"("refnum name"="navX") -> ("navX Device"=w260:T4)  [unwired: 9 in, 1 out]
          n174 = call <vilib>:"WPI_EncoderRefNum Registry Get.vi"("refnum name"="Encoder 2") -> ("EncoderDevRef"=w262:T6)  [unwired: 9 in, 1 out]
          n175 = call <vilib>:"WPI_EncoderRefNum Registry Get.vi"("refnum name"="Encoder 1") -> ("EncoderDevRef"=w264:T6)  [unwired: 9 in, 1 out]
          n176 = call "Z900_navX_Set_ZeroYaw.vi"("navX Device"=w260) -> ("navX Device"=w259:T4)  [unwired: 9 in, 1 out]
          n177 = call <vilib>:"WPI_EncoderReset.vi"("EncoderDevRef"=w262) -> ("EncoderDevRef"=w261:T6)  [unwired: 9 in, 1 out]
          n178 = call <vilib>:"WPI_EncoderReset.vi"("EncoderDevRef"=w264) -> ("EncoderDevRef"=w263:T6)  [unwired: 9 in, 1 out]
          n179 = while {
            tunnel: w263 -> [_]
            tunnel: w261 -> [_]
            tunnel: w259 -> [w278]
            stop <- w272 stop-if-true
            n180 = call "Z900_navX_Get_YPRHfH.vi"("navX Device"=w278) -> ("YRPHfH"=w277:T10)  [unwired: 7 in, 3 out]
            n181 = call-poly <vilib>:"NT Read Value.vi"("Name"="Position") -> ("Numeric"=w269:dbl)  [unwired: 9 in, 1 out]
            n182 = case shown="Default" w269 {
              tunnel: [0.0 35.0 20.0 0.0 -20.0 -45.0] -> w270
              frame Default {
              }
              frame 1 {
              }
              frame 2 {
              }
              frame 3 {
              }
              frame 4 {
              }
              frame 5 {
              }
            }
            n183 = Unbundle By Name(w277) -> ("Yaw"=w275:dbl)  [unwired: 1 out]
            n184 = local read "Single Turn Gains"() -> (w268:T1)
            n185 = call-poly <vilib>:"PID.vi"("output range"=cluster{"output high":dbl, "output low":dbl} {"output high"=0.8, "output low"=-0.8}, "PID gains"=w268, "process variable"=w275, "setpoint"=w270) -> ("output"=w274:dbl)  [unwired: 6 in, 1 out]
            n186 = Multiply(x=-1.0, y=w274) -> (x*y=w273:dbl)
            n187 = call <vilib>:"WPI_RobotDriveRefNum Registry Get.vi"("refnum name"="Left and Right Motors") -> ("RobotDriveDevRef"=w281:T11)  [unwired: 9 in, 1 out]
            n188 = call <vilib>:"WPI_RobotDriveTankDrive.vi"("Right axis value"=w274, "Left axis value"=w273, "RobotDriveDevRef"=w281) -> ()  [unwired: 6 in, 3 out]
            n189 = call "Elapsed Time3"() -> ("Time has Elapsed"=w272:bool)  [unwired: 12 in, 7 out]
            n190 = Wait (ms)(milliseconds to wait=u32 50) -> ()  [unwired: 1 out]
          }
        }
      }
    }
    frame "New 2-Ball" {
      n191 = flat-sequence {
        frame #0 {
          w289 = u16 6 items=["Forward", "Backward", "Turn", "Shoot", "Turn Angle", "Roll G", "Roll L"] ("Task")
          n192 = call "Auton Commands.vi"("Roll"=-5.0, "Turn Angle"=0.0, "Distance"=120.0, "Task"=w289) -> ()  [unwired: 7 in]
        }
        frame #1 {
          w293 = u16 5 items=["Forward", "Backward", "Turn", "Shoot", "Turn Angle", "Roll G", "Roll L"] ("Task")
          n193 = call "Auton Commands.vi"("Roll"=-3.0, "Turn Angle"=0.0, "Distance"=120.0, "Task"=w293) -> ()  [unwired: 7 in]
        }
        frame #2 {
          w297 = u16 0 items=["Forward", "Backward", "Turn", "Shoot", "Turn Angle", "Roll G", "Roll L"] ("Task")
          n194 = call "Auton Commands.vi"("Roll"=0.0, "Turn Angle"=0.0, "Distance"=120.0, "Task"=w297) -> ()  [unwired: 7 in]
        }
        frame #3 {
          w301 = u16 2 items=["Forward", "Backward", "Turn", "Shoot", "Turn Angle", "Roll G", "Roll L"] ("Task")
          n195 = call "Auton Commands.vi"("Roll"=0.0, "Turn Angle"=0.0, "Distance"=120.0, "Task"=w301) -> ()  [unwired: 7 in]
        }
        frame #4 {
          w305 = u16 3 items=["Forward", "Backward", "Turn", "Shoot", "Turn Angle", "Roll G", "Roll L"] ("Task")
          n196 = call "Auton Commands.vi"("Roll"=0.0, "Turn Angle"=0.0, "Distance"=120.0, "Task"=w305) -> ()  [unwired: 7 in]
        }
        frame #5 {
          w309 = u16 4 items=["Forward", "Backward", "Turn", "Shoot", "Turn Angle", "Roll G", "Roll L"] ("Task")
          n197 = call "Auton Commands.vi"("Roll"=0.0, "Turn Angle"=150.0, "Distance"=120.0, "Task"=w309) -> ()  [unwired: 7 in]
        }
        frame #6 {
          w313 = u16 0 items=["Forward", "Backward", "Turn", "Shoot", "Turn Angle", "Roll G", "Roll L"] ("Task")
          n198 = call "Auton Commands.vi"("Roll"=0.0, "Turn Angle"=0.0, "Distance"=120.0, "Task"=w313) -> ()  [unwired: 7 in]
        }
        frame #7 {
          w317 = u16 6 items=["Forward", "Backward", "Turn", "Shoot", "Turn Angle", "Roll G", "Roll L"] ("Task")
          n199 = call "Auton Commands.vi"("Roll"=-5.0, "Turn Angle"=0.0, "Distance"=120.0, "Task"=w317) -> ()  [unwired: 7 in]
        }
        frame #8 {
          w321 = u16 5 items=["Forward", "Backward", "Turn", "Shoot", "Turn Angle", "Roll G", "Roll L"] ("Task")
          n200 = call "Auton Commands.vi"("Roll"=-3.0, "Turn Angle"=0.0, "Distance"=120.0, "Task"=w321) -> ()  [unwired: 7 in]
        }
        frame #9 {
          w325 = u16 0 items=["Forward", "Backward", "Turn", "Shoot", "Turn Angle", "Roll G", "Roll L"] ("Task")
          n201 = call "Auton Commands.vi"("Roll"=0.0, "Turn Angle"=0.0, "Distance"=60.0, "Task"=w325) -> ()  [unwired: 7 in]
        }
        frame #10 {
          w329 = u16 1 items=["Forward", "Backward", "Turn", "Shoot", "Turn Angle", "Roll G", "Roll L"] ("Task")
          n202 = call "Auton Commands.vi"("Roll"=0.0, "Turn Angle"=0.0, "Distance"=180.0, "Task"=w329) -> ()  [unwired: 7 in]
        }
        frame #11 {
          w333 = u16 4 items=["Forward", "Backward", "Turn", "Shoot", "Turn Angle", "Roll G", "Roll L"] ("Task")
          n203 = call "Auton Commands.vi"("Roll"=0.0, "Turn Angle"=-150.0, "Distance"=180.0, "Task"=w333) -> ()  [unwired: 7 in]
        }
        frame #12 {
          w337 = u16 3 items=["Forward", "Backward", "Turn", "Shoot", "Turn Angle", "Roll G", "Roll L"] ("Task")
          n204 = call "Auton Commands.vi"("Roll"=0.0, "Turn Angle"=-150.0, "Distance"=180.0, "Task"=w337) -> ()  [unwired: 7 in]
        }
      }
    }
    frame "Drive + Shoot" {
      n205 = call "Z900_navX_RefNum_Get.vi"("refnum name"="navX") -> ("navX Device"=w349:T4)  [unwired: 9 in, 1 out]
      n206 = call <vilib>:"WPI_EncoderRefNum Registry Get.vi"("refnum name"="Encoder 2") -> ("EncoderDevRef"=w347:T6)  [unwired: 9 in, 1 out]
      n207 = call <vilib>:"WPI_EncoderRefNum Registry Get.vi"("refnum name"="Encoder 1") -> ("EncoderDevRef"=w345:T6)  [unwired: 9 in, 1 out]
      n208 = call "Z900_navX_Set_ZeroYaw.vi"("navX Device"=w349) -> ("navX Device"=w350:T4)  [unwired: 9 in, 1 out]
      n209 = call <vilib>:"WPI_EncoderReset.vi"("EncoderDevRef"=w347) -> ("EncoderDevRef"=w348:T6)  [unwired: 9 in, 1 out]
      n210 = call <vilib>:"WPI_EncoderReset.vi"("EncoderDevRef"=w345) -> ("EncoderDevRef"=w346:T6)  [unwired: 9 in, 1 out]
      n211 = flat-sequence {
        tunnel: w350 -> [w354]
        tunnel: w348 -> [w353]
        tunnel: w346 -> [w352]
        tunnel: w341 -> [w351]
        frame #0 {
          n212 = while {
            tunnel: w352 -> [w392]
            tunnel: w353 -> [w391]
            tunnel: w354 -> [w390]
            tunnel: w351 -> [w360]
            stop <- w361 stop-if-true
            n213 = call <vilib>:"WPI_EncoderGet.vi"("EncoderDevRef"=w391) -> ("Distance"=w367:dbl, "Rate"=→"E2 Rate":dbl)  [unwired: 5 in, 4 out]
            n214 = call-poly <vilib>:"NT Read Value.vi"("Name"=w360) -> ("Numeric"=w359:dbl)  [unwired: 9 in, 1 out]
            n215 = call "Z900_navX_Get_YPRHfH.vi"("navX Device"=w390) -> ("YRPHfH"=w393:T10)  [unwired: 7 in, 3 out]
            n216 = Divide(x=w359, y=100.0) -> (x/y=w357:dbl)
            n217 = call <vilib>:"WPI_EncoderGet.vi"("EncoderDevRef"=w392) -> ("Distance"=w368:dbl, "Rate"=→"E1 Rate":dbl)  [unwired: 5 in, 4 out]
            n218 = Bundle(w357, "output low"=0.15) -> (w355:cluster{dbl, "output low":dbl})  [unwired: 1 in]
            n219 = Unbundle By Name(w393) -> ("Yaw"=w369:dbl)  [unwired: 1 out]
            "Yaw" <- w369
            n220 = call-poly <vilib>:"NT Write Value.vi"("Numeric"=w367, "Name"="E2 Dist") -> ()  [unwired: 9 in, 1 out]
            n221 = local read "Distance"() -> (w377:dbl)
            n222 = call-poly <vilib>:"NT Write Value.vi"("Numeric"=w368, "Name"="E1 Dist") -> ()  [unwired: 9 in, 1 out]
            n223 = Multiply(x=w377, y=13.7) -> (x*y=w366:dbl)
            n224 = local read "Speed Gains"() -> (w371:T1)
            n225 = local read "Yaw"() -> (w375:T1)
            n226 = Add(x=w368, y=w367) -> (x+y=w389:dbl)
            n227 = Divide(x=w389, y=2.0) -> (x/y=w365:dbl)
            n228 = Subtract(x=w366, y=w365) -> (x-y=w364:dbl)
            n229 = Absolute Value(x=w364) -> (abs(x)=w363:dbl)
            n230 = Less?(x=w363, y=30.0) -> (x < y?=w361:bool)
            n231 = call-poly <vilib>:"PID.vi"("output range"=cluster{"output high":dbl, "output low":dbl} {"output high"=0.2, "output low"=-0.2}, "PID gains"=w375, "process variable"=w369, "setpoint"=0.0) -> ("output"=w382:dbl)  [unwired: 6 in, 1 out]
            n232 = call-poly <vilib>:"PID.vi"("output range"=w355, "PID gains"=w371, "process variable"=w365, "setpoint"=w366) -> ("output"=w379:dbl)  [unwired: 6 in, 1 out]
            n233 = Multiply(x=-1.0, y=w382) -> (x*y=w383:dbl)
            n234 = Add(x=1.0, y=w383) -> (x+y=w384:dbl)
            n235 = Wait (ms)(milliseconds to wait=u32 50) -> ()  [unwired: 1 out]
            n236 = Add(x=w382, y=1.0) -> (x+y=w385:dbl)
            n237 = Multiply(x=w379, y=w384) -> (x*y=w372:dbl)
            n238 = Multiply(x=w379, y=w385) -> (x*y=w374:dbl)
            n239 = call <vilib>:"WPI_RobotDriveRefNum Registry Get.vi"("refnum name"="Left and Right Motors") -> ("RobotDriveDevRef"=w395:T11)  [unwired: 9 in, 1 out]
            n240 = call <vilib>:"WPI_RobotDriveTankDrive.vi"("Right axis value"=w374, "Left axis value"=w372, "RobotDriveDevRef"=w395) -> ()  [unwired: 6 in, 3 out]
            n241 = local write "Right Motor Speed"(w374) -> ()
            n242 = local write "Left Motor Speed"(w372) -> ()
          }
        }
        frame #1 {
          n243 = call "Z900_navX_RefNum_Get.vi"("refnum name"="navX") -> ("navX Device"=w400:T4)  [unwired: 9 in, 1 out]
          n244 = call <vilib>:"WPI_EncoderRefNum Registry Get.vi"("refnum name"="Encoder 2") -> ("EncoderDevRef"=w402:T6)  [unwired: 9 in, 1 out]
          n245 = call <vilib>:"WPI_EncoderRefNum Registry Get.vi"("refnum name"="Encoder 1") -> ("EncoderDevRef"=w404:T6)  [unwired: 9 in, 1 out]
          n246 = call "Z900_navX_Set_ZeroYaw.vi"("navX Device"=w400) -> ("navX Device"=w399:T4)  [unwired: 9 in, 1 out]
          n247 = call <vilib>:"WPI_EncoderReset.vi"("EncoderDevRef"=w402) -> ("EncoderDevRef"=w401:T6)  [unwired: 9 in, 1 out]
          n248 = call <vilib>:"WPI_EncoderReset.vi"("EncoderDevRef"=w404) -> ("EncoderDevRef"=w403:T6)  [unwired: 9 in, 1 out]
          n249 = while {
            tunnel: w403 -> [_]
            tunnel: w401 -> [_]
            tunnel: w399 -> [w418]
            stop <- w411 stop-if-true
            n250 = call "Z900_navX_Get_YPRHfH.vi"("navX Device"=w418) -> ("YRPHfH"=w417:T10)  [unwired: 7 in, 3 out]
            n251 = call-poly <vilib>:"NT Read Value.vi"("Name"="Position") -> ("Numeric"=w408:dbl)  [unwired: 9 in, 1 out]
            n252 = case shown="Default" w408 {
              tunnel: [0.0 35.0 20.0 0.0 -20.0 -45.0] -> w409
              frame Default {
              }
              frame 1 {
              }
              frame 2 {
              }
              frame 3 {
              }
              frame 4 {
              }
              frame 5 {
              }
            }
            n253 = Unbundle By Name(w417) -> ("Yaw"=w415:dbl)  [unwired: 1 out]
            n254 = local read "Single Turn Gains"() -> (w414:T1)
            n255 = call-poly <vilib>:"PID.vi"("output range"=cluster{"output high":dbl, "output low":dbl} {"output high"=0.8, "output low"=-0.8}, "PID gains"=w414, "process variable"=w415, "setpoint"=w409) -> ("output"=w413:dbl)  [unwired: 6 in, 1 out]
            n256 = local write "Left Motor Speed"(w413) -> ()
            n257 = Multiply(x=-1.0, y=w413) -> (x*y=w412:dbl)
            n258 = local write "Right Motor Speed"(w412) -> ()
            n259 = call <vilib>:"WPI_RobotDriveRefNum Registry Get.vi"("refnum name"="Left and Right Motors") -> ("RobotDriveDevRef"=w421:T11)  [unwired: 9 in, 1 out]
            n260 = call <vilib>:"WPI_RobotDriveTankDrive.vi"("Right axis value"=w413, "Left axis value"=w412, "RobotDriveDevRef"=w421) -> ()  [unwired: 6 in, 3 out]
            n261 = call "Elapsed Time"() -> ("Time has Elapsed"=w411:bool)  [unwired: 12 in, 7 out]
            n262 = Wait (ms)(milliseconds to wait=u32 50) -> ()  [unwired: 1 out]
          }
        }
        frame #2 {
          n263 = while {
            stop <- w439 stop-if-true
            n264 = local read "Aiming Gains"() -> (w429:T1)
            n265 = global read "Robot Global Data.vi" "T1 X"() -> (w437:dbl)
            n266 = Absolute Value(x=w437) -> (abs(x)=w442:dbl)
            n267 = Less?(x=w442, y=0.05) -> (x < y?=w440:bool)
            n268 = call-poly <vilib>:"PID.vi"("output range"=cluster{"output high":dbl, "output low":dbl} {"output high"=0.7, "output low"=-0.7}, "PID gains"=w429, "process variable"=w437, "setpoint"=0.0) -> ("output"=w431:dbl)  [unwired: 6 in, 1 out]
            n269 = case shown="False" w440 {
              tunnel: [FALSE FALSE] -> w439
              frame False {
              }
              frame True {
              }
            }
            n270 = Multiply(x=w431, y=-1.0) -> (x*y=w430:dbl)
            n271 = call <vilib>:"WPI_RobotDriveRefNum Registry Get.vi"("refnum name"="Left and Right Motors") -> ("RobotDriveDevRef"=w433:T11)  [unwired: 9 in, 1 out]
            n272 = call <vilib>:"WPI_RobotDriveTankDrive.vi"("Right axis value"=w430, "Left axis value"=w431, "RobotDriveDevRef"=w433) -> ()  [unwired: 6 in, 3 out]
            n273 = Wait (ms)(milliseconds to wait=u32 50) -> ()  [unwired: 1 out]
          }
        }
      }
    }
    frame "Dashboard Auton" {
      n274 = flat-sequence {
        frame #0 {
          n275 = while {
            stop <- w455 stop-if-true
            n276 = global read "Robot Global Data.vi" "T1 X"() -> (w453:dbl)
            n277 = Absolute Value(x=w453) -> (abs(x)=w458:dbl)
            n278 = Less?(x=w458, y=0.05) -> (x < y?=w456:bool)
            n279 = call-poly <vilib>:"PID.vi"("output range"=cluster{"output high":dbl, "output low":dbl} {"output high"=0.7, "output low"=-0.7}, "PID gains"="Aiming Gains", "process variable"=w453, "setpoint"=0.0) -> ("output"=w446:dbl)  [unwired: 6 in, 1 out]
            n280 = case shown="False" w456 {
              tunnel: [FALSE FALSE] -> w455
              frame False {
              }
              frame True {
              }
            }
            n281 = Multiply(x=w446, y=-1.0) -> (x*y=w445:dbl)
            n282 = call <vilib>:"WPI_RobotDriveRefNum Registry Get.vi"("refnum name"="Left and Right Motors") -> ("RobotDriveDevRef"=w448:T11)  [unwired: 9 in, 1 out]
            n283 = call <vilib>:"WPI_RobotDriveTankDrive.vi"("Right axis value"=w445, "Left axis value"=w446, "RobotDriveDevRef"=w448) -> ()  [unwired: 6 in, 3 out]
            n284 = Wait (ms)(milliseconds to wait=u32 50) -> ()  [unwired: 1 out]
          }
        }
      }
    }
  }
